vi "Cubic Motion Profile.vi"(7 "Reset?":bool, 11 "Distance":dbl) -> (3 "Y Throttle":dbl, 4 "Profile Complete?":bool)   [LabVIEW 2015]
uses:
  <vilib>/Rock Robotics/Network Tables/NT Read Number.vi
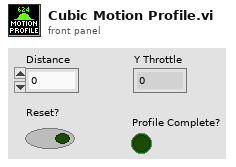
[diagram p1: front panel]
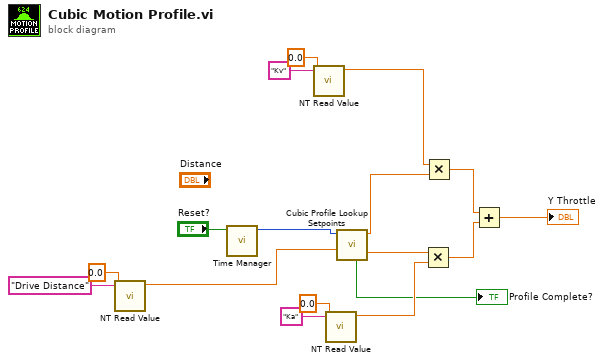
[diagram p0: block diagram]
diagram:
  n1 = call-poly <vilib>:"NT Read Value.vi"("Default Value"=0.0, "Name"="Drive Distance") -> ("Numeric"=w2:dbl)  [unwired: 8 in, 1 out]
  n2 = call "Time Manager.vi"("Reset?"="Reset?") -> ("Elapsed Time"=w13:u32)  [unwired: 10 in]
  n3 = call-poly <vilib>:"NT Read Value.vi"("Default Value"=0.0, "Name"="Kv") -> ("Numeric"=w14:dbl)  [unwired: 8 in, 1 out]
  n4 = call-poly <vilib>:"NT Read Value.vi"("Default Value"=0.0, "Name"="Ka") -> ("Numeric"=w8:dbl)  [unwired: 8 in, 1 out]
  n5 = call "Cubic Profile Lookup Setpoints.vi"("Distance"=w2, "Current Time"=w13) -> ("Acceleration"=w11:dbl, "Velocity"=w12:dbl, "Complete?"=→"Profile Complete?":bool)  [unwired: 7 in]
  n6 = Multiply(x=w11, y=w8) -> (x*y=w6:dbl)
  n7 = Multiply(x=w14, y=w12) -> (x*y=w7:dbl)
  n8 = Add(x=w7, y=w6) -> (x+y=→"Y Throttle":dbl)
